vi "ReadMultimeterVoltage.vi"(8 "error in (no error)":errorcluster, 11 "MultimeterSim in":refnum<class "MultimeterSim.lvclass">) -> (0 "error out":errorcluster, 2 "Voltage":dbl, 3 "MultimeterSim out":refnum<class "MultimeterSim.lvclass">)   [LabVIEW 2017, in "MultimeterSim.lvclass"]
uses:
  MultimeterSim.lvclass
  MultimeterSim.lvclass/MultimeterSim.ctl
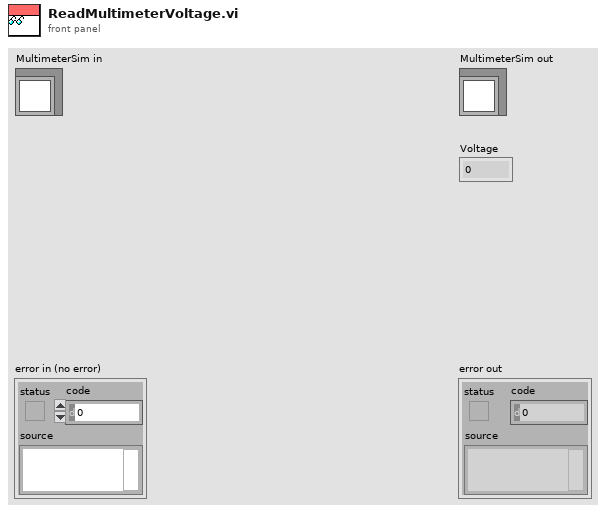
[diagram p1: front panel]
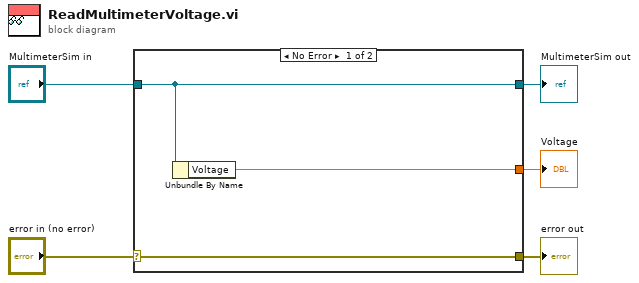
[diagram p0: block diagram]
diagram:
  n1 = case shown="No Error" "error in (no error)" {
    selector: "error in (no error)" -> [w8 w9]
    tunnel: [w8 w9] -> w4
    tunnel: [w7 w10] -> w2
    tunnel: "MultimeterSim in" -> [w7 w10]
    tunnel: [w6 _] -> w1
    frame No Error {
      n2 = Unbundle By Name(w7) -> ("Voltage"=w6:dbl)
    }
    frame Error {
    }
  }
  "error out" <- w4
  "MultimeterSim out" <- w2
  "Voltage" <- w1
